vi "Send Receive.vi"(8 "Error In":errorcluster, 9 "Bytes To Read":u32, 10 "Packet":string, 11 "EZ430-Chronos Config":T1) -> (0 "Error Out":errorcluster, 2 "Data":u8[](array[numeric]), 3 "EZ430-Chronos Config":T1)   [LabVIEW 2011, in "LVH-EZ430.lvlib"]
doc: "Send a command to the EZ430-Chronos and read the response."
uses:
  LVH-EZ430.lvlib
  Type Defs/EZ430-Chronos Ref.ctl
panel:
  in  "Retries":u32=10
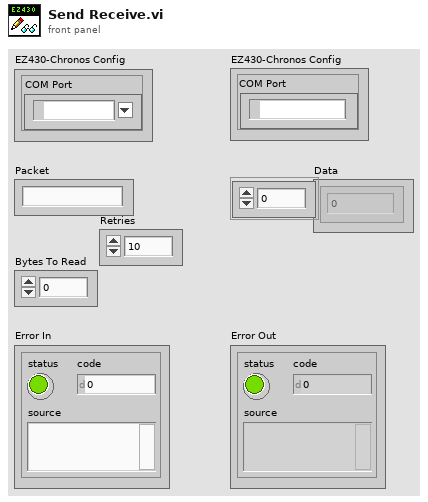
[diagram p1: front panel]
types:
  T1 = typedef "LVH-EZ430.lvlib/EZ430-Chronos Ref.ctl" = cluster{"COM Port":refnum<visa-resource-name>}
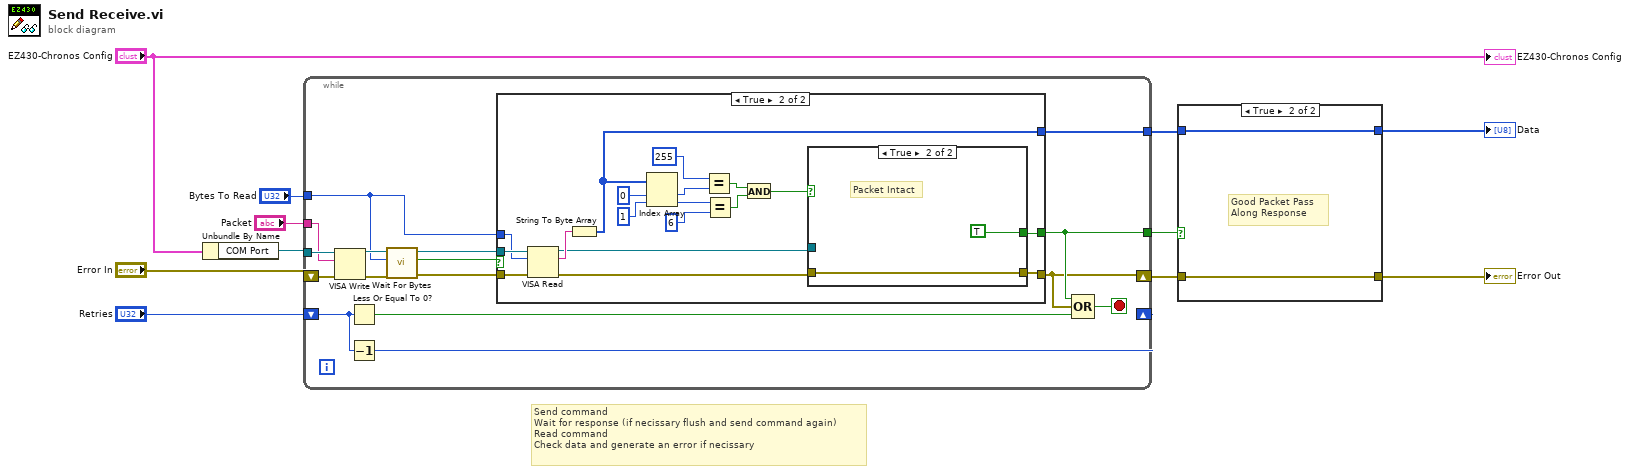
[diagram p0: block diagram]
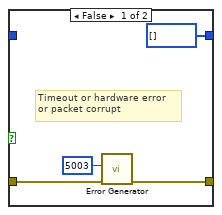
[diagram p2: hidden frame]
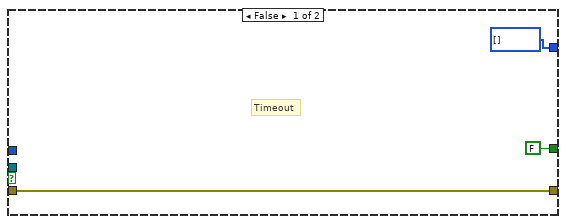
[diagram p3: hidden frame]
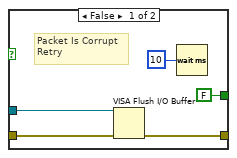
[diagram p4: hidden frame]
diagram:
  # "Send command\nWait for response (if necissary flush and send command again)\nRead command\nCheck data and generate an error if necissary"
  n1 = Unbundle By Name("EZ430-Chronos Config") -> ("COM Port"=w7:refnum<visa-resource-name>)
  n2 = while {
    shift-right: [w26] -> _
    shift-left: "Retries" -> [w27]
    tunnel: w7 -> [w24]
    tunnel: "Bytes To Read" -> [w17]
    shift-right: [w14] -> w3
    shift-left: "Error In" -> [w23]
    tunnel: [w15] -> w4
    tunnel: [w16] -> w2
    tunnel: "Packet" -> [w13]
    stop <- w25 stop-if-true
    n3 = VISA Write(VISA resource name=w24, write buffer=w13, error in (no error)=w23) -> (VISA resource name out=w21:refnum<visa-resource-name>, error out=w22:errorcluster)  [unwired: 1 out]
    n4 = Less Or Equal To 0?(x=w27) -> (x <= 0?=w12:bool)
    n5 = Decrement(x=w27) -> (x-1=w26:u32)
    n6 = call "Wait For Bytes.vi"("Error In"=w22, "Bytes To Read"=w17, "VISA resource name"=w21) -> ("Error Out"=w19:errorcluster, "Bytes Available?"=w20:bool, "VISA resource name"=w18:refnum<visa-resource-name>)  [unwired: 6 in]
    n7 = case shown="True" w20 {
      tunnel: w19 -> [w29 w48]
      tunnel: w18 -> [_ w47]
      tunnel: w17 -> [_ w46]
      tunnel: [FALSE w41] -> w15
      tunnel: [w29 w38] -> w14
      tunnel: [u8[] [] ("unsigned byte array") w37] -> w16
      frame False {
        # "Timeout"
      }
      frame True {
        n8 = VISA Read(VISA resource name=w47, byte count=w46, error in (no error)=w48) -> (VISA resource name out=w40:refnum<visa-resource-name>, read buffer=w43:string, error out=w39:errorcluster)  [unwired: 1 out]
        n9 = String To Byte Array(string=w43) -> (unsigned byte array=w37:u8[])
        n10 = Index Array(array=w37, index #1=0 ("index"), index #2=1 ("index")) -> (element #1=w42:u8, element #2=w32:u8)
        n11 = Equal?(x=u8 255, y=w42) -> (x = y?=w34:bool)
        n12 = Equal?(x=w32, y=u8 6 ("x")) -> (x = y?=w35:bool)
        n13 = And(x=w34, y=w35) -> (x .and. y?=w31:bool)
        n14 = case shown="True" w31 {
          tunnel: [FALSE TRUE] -> w41
          tunnel: w40 -> [w52 _]
          tunnel: w39 -> [w51 w54]
          tunnel: [w50 w54] -> w38
          frame False {
            # "Packet Is Corrupt\nRetry"
            n15 = VISA Flush I/O Buffer(VISA resource name=w52, error in (no error)=w51) -> (error out=w50:errorcluster)  [unwired: 1 in, 1 out]
            n16 = Wait (ms)(milliseconds to wait=u32 10) -> ()  [unwired: 1 out]
          }
          frame True {
            # "Packet Intact"
          }
        }
      }
    }
    n17 = Compound Arithmetic op=OR(w15, w14, w12) -> (w25:bool)
  }
  n18 = case shown="True" w4 {
    tunnel: [w58 w61] -> w10
    tunnel: w3 -> [w59 w61]
    tunnel: [u8[] [] ("unsigned byte array") w60] -> w9
    tunnel: w2 -> [_ w60]
    frame False {
      # "Timeout or hardware error \nor packet corrupt"
      n19 = call "Error Generator.vi"("Error In"=w59, "EZ430-Chronos Error Code"=5003) -> ("Error Out"=w58:errorcluster)  [unwired: 8 in, 1 out]
    }
    frame True {
      # "Good Packet Pass \nAlong Response"
    }
  }
  "Error Out" <- w10
  "Data" <- w9
  "EZ430-Chronos Config" <- "EZ430-Chronos Config"
